vi "GUI De-Init.vi"(8 "error in (no error)":errorcluster, 10 "GUI Refs":T1, 11 "View Model":T2) -> (0 "error out":errorcluster, 3 "View Model":T2)   [LabVIEW 2017]
doc: "De - Initialize all GUI Arrays of all used modules\nMake array's size equal to 1 element values = empty"
uses:
  View Model/Controls/View Model.ctl
  View Model/Controls/Shared Model.ctl
  Error Handler/Controls/Error Model.ctl
  Error Handler/Controls/Error Event.ctl
  Error Handler/Controls/Error Type.ctl
  Controller/Controls/Controller Model.ctl
  Controller/Controls/Controller Event.ctl
  Controller/Controls/Controller Command.ctl
  Controller/Controls/Controller Overhead.ctl
  Real-Time/RT Status.ctl
  Real-Time/RT Loop Status.ctl
  Controller/Controls/Controller DAQ Data.ctl
  Controls/GUI Referencies.ctl
  Controls/AIMV_GUI_Cluster.ctl
  Controls/AOM_GUI_Cluster.ctl
  Controls/Discrete_GUI_Cluster.ctl
  GUI Init - AIMC.vi
  GUI Init - AIMV.vi
  GUI Init - AOM.vi
  GUI Init - DIM.vi
  GUI Init - DOM.vi
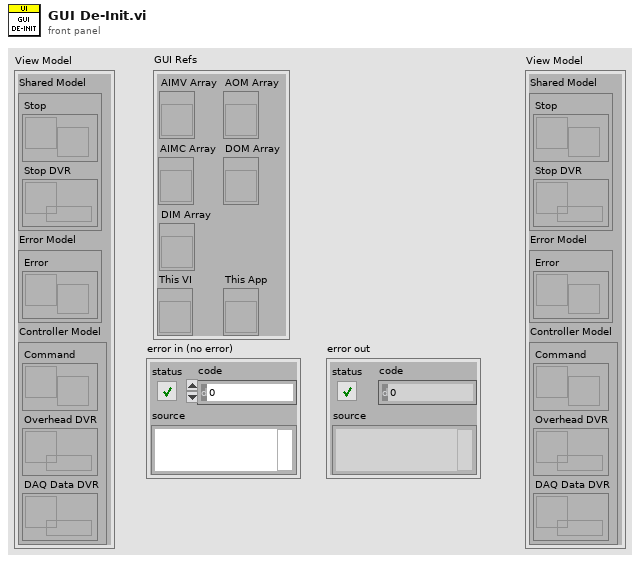
[diagram p1: front panel]
types:
  T1 = typedef "GUI Referencies.ctl" = cluster{"AIMV Array":refnum<vi>, "AIMC Array":refnum<vi>, "AOM Array":refnum<vi>, "DIM Array":refnum<vi>, "DOM Array":refnum<vi>, "This VI":refnum<vi>, "This App":refnum<vi>}
  T2 = typedef "View Model.ctl" = cluster{"Shared Model":T3, "Error Model":T4, "Controller Model":T5}
  T3 = typedef "Shared Model.ctl" = cluster{"Stop":refnum<user-event>, "Stop DVR":refnum<data-value>}
  T4 = typedef "Error Model.ctl" = cluster{"Error":refnum<user-event>}
  T5 = typedef "Controller Model.ctl" = cluster{"Command":refnum<user-event>, "Overhead DVR":refnum<data-value>, "DAQ Data DVR":refnum<data-value>}
  T6 = enum8{"Enabled", "Disabled", "Disabled and Grayed Out"}
  T7 = typedef "Controller DAQ Data.ctl" = cluster{"AOM data":dbl[], "AIMV data":dbl[], "AIMC data":dbl[], "DOM data":dbl[], "DIM data":dbl[], "AOM timestamp":dbl, "AIMV timestamp":dbl, "AIMC timestamp":dbl, "DOM timestamp":dbl, "DIM timestamp":dbl}
  T8 = typedef "AIMV_GUI_Cluster.ctl" = cluster{"Ch.name":string, "Ch.value":dbl, "Ch.range":string}
  T9 = typedef "Discrete_GUI_Cluster.ctl" = cluster{"Ch.name":string, "Ch.state":bool}
  T10 = typedef "AOM_GUI_Cluster.ctl" = cluster{"Ch.name":string, "Ch.value":dbl, "Ch.mode":enum16{"0-5 V", "+/-10 V", "0-5 mA", "4-20 mA"}}
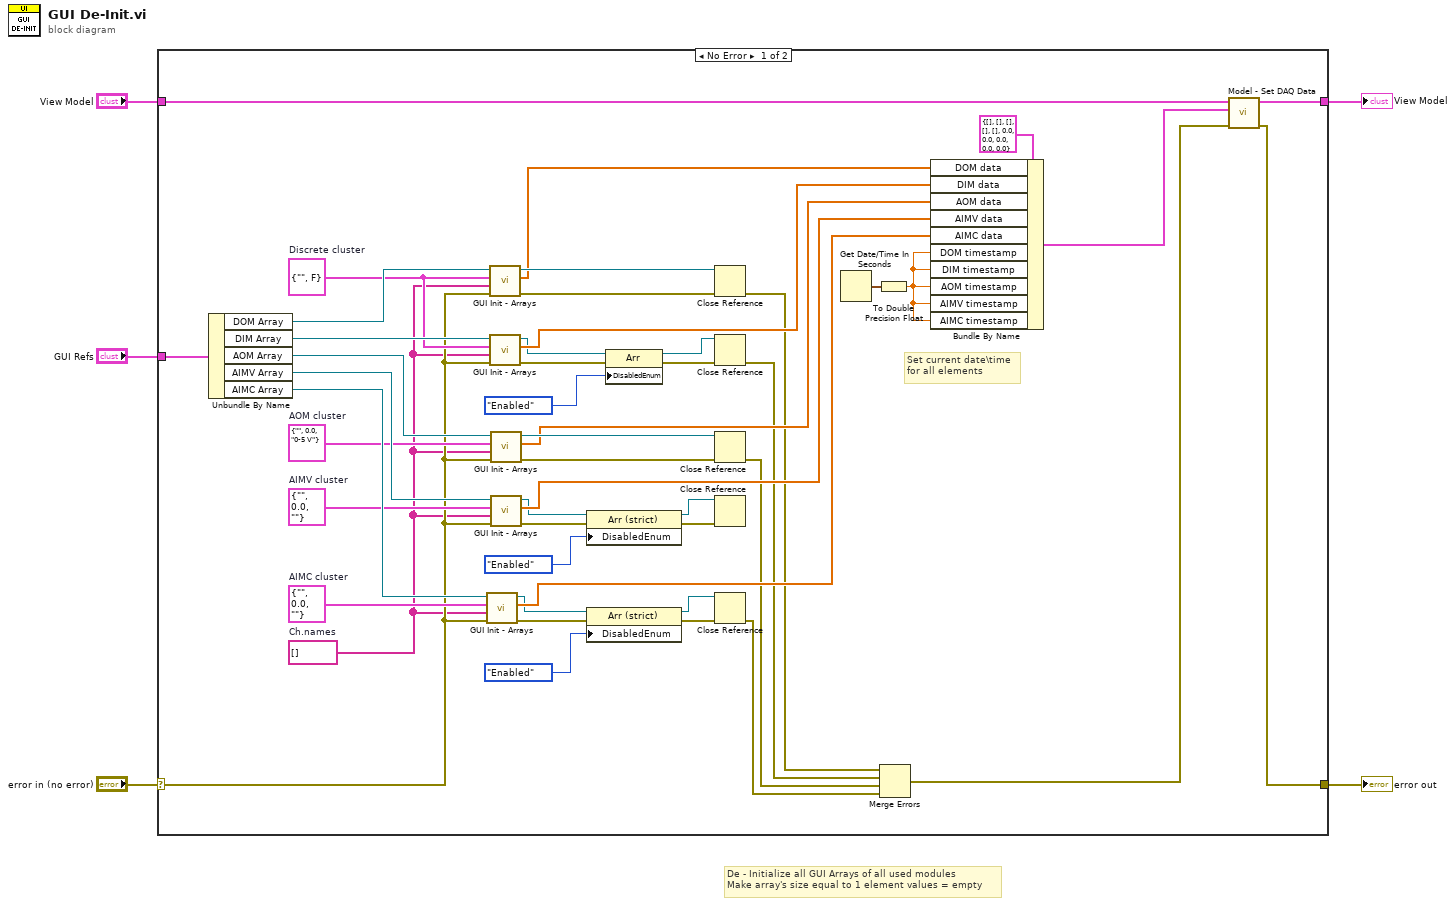
[diagram p0: block diagram]
diagram:
  # "De - Initialize all GUI Arrays of all used modules\nMake array's size equal to 1 element values = empty"
  n1 = case shown="No Error" "error in (no error)" {
    selector: "error in (no error)" -> [w43 w54]
    tunnel: [w35 w54] -> w4
    tunnel: "View Model" -> [w39 w55]
    tunnel: [w37 w55] -> w2
    tunnel: "GUI Refs" -> [w53 _]
    frame No Error {
      w45 = T8 {"Ch.name"="", "Ch.value"=0.0, "Ch.range"=""}  # AIMV cluster
      w34 = string[] []  # Ch.names
      w47 = T9 {"Ch.name"="", "Ch.state"=FALSE}  # Discrete cluster
      w46 = T10 {"Ch.name"="", "Ch.value"=0.0, "Ch.mode"=enum."0-5 V"}  # AOM cluster
      w44 = T8 {"Ch.name"="", "Ch.value"=0.0, "Ch.range"=""}  # AIMC cluster
      # "Set current date\\time\nfor all elements"
      n2 = Unbundle By Name(w53) -> ("DOM Array"=w52:refnum<vi>, "DIM Array"=w51:refnum<vi>, "AOM Array"=w50:refnum<vi>, "AIMV Array"=w49:refnum<vi>, "AIMC Array"=w48:refnum<vi>)
      n3 = call-poly "GUI Init - Arrays.vi"("error in (no error)"=w43, "Ch.names"=w34, "Cluster"=w44, "Array Ref."=w48) -> ("error out"=w18:errorcluster, "Data"=w29:dbl[], "Array Ref. out"=w9:refnum<vi>)  [unwired: 5 in]
      n4 = call-poly "GUI Init - Arrays.vi"("error in (no error)"=w43, "Ch.names"=w34, "Cluster"=w47, "Array Ref."=w52) -> ("error out"=w33:errorcluster, "Data"=w25:dbl[], "Array Ref. out"=w32:refnum<vi>)  [unwired: 5 in]
      n5 = call-poly "GUI Init - Arrays.vi"("error in (no error)"=w43, "Ch.names"=w34, "Cluster"=w47, "Array Ref."=w51) -> ("error out"=w20:errorcluster, "Data"=w26:dbl[], "Array Ref. out"=w7:refnum<vi>)  [unwired: 5 in]
      n6 = call-poly "GUI Init - Arrays.vi"("error in (no error)"=w43, "Ch.names"=w34, "Cluster"=w46, "Array Ref."=w50) -> ("error out"=w31:errorcluster, "Data"=w27:dbl[], "Array Ref. out"=w30:refnum<vi>)  [unwired: 5 in]
      n7 = call-poly "GUI Init - Arrays.vi"("error in (no error)"=w43, "Ch.names"=w34, "Cluster"=w45, "Array Ref."=w49) -> ("error out"=w16:errorcluster, "Data"=w28:dbl[], "Array Ref. out"=w11:refnum<vi>)  [unwired: 5 in]
      n8 = property class="Arr (strict)"(reference=w11, error in=w16, "DisabledEnum"=T6."Enabled" ("Disabled")) -> (reference out=w10:refnum<vi>, error out=w15:errorcluster)
      n9 = property class="Arr (strict)"(reference=w9, error in=w18, "DisabledEnum"=T6."Enabled" ("Disabled")) -> (reference out=w8:refnum<vi>, error out=w17:errorcluster)
      n10 = property class="Arr"(reference=w7, error in=w20, "DisabledEnum"=T6."Enabled" ("Disabled")) -> (reference out=w6:refnum<vi>, error out=w19:errorcluster)
      n11 = Close Reference(reference=w32, error in (no error)=w33) -> (error out=w24:errorcluster)
      n12 = Close Reference(reference=w6, error in (no error)=w19) -> (error out=w23:errorcluster)
      n13 = Close Reference(reference=w30, error in (no error)=w31) -> (error out=w22:errorcluster)
      n14 = Close Reference(reference=w10, error in (no error)=w15) -> ()  [unwired: 1 out]
      n15 = Close Reference(reference=w8, error in (no error)=w17) -> (error out=w21:errorcluster)
      n16 = Get Date/Time In Seconds() -> (seconds since 1Jan1904=w41:timestamp)
      n17 = To Double Precision Float(number=w41) -> (double precision float=w40:dbl)
      n18 = Merge Errors(w24, w23, w22, w21) -> (w36:errorcluster)
      n19 = Bundle By Name(cluster=T7 {"AOM data"=[], "AIMV data"=[], "AIMC data"=[], "DOM data"=[], "DIM data"=[], "AOM timestamp"=0.0, "AIMV timestamp"=0.0, "AIMC timestamp"=0.0, "DOM timestamp"=0.0, "DIM timestamp"=0.0} ("DAQ Data"), "DOM data"=w25, "DIM data"=w26, "AOM data"=w27, "AIMV data"=w28, "AIMC data"=w29, "DOM timestamp"=w40, "DIM timestamp"=w40, "AOM timestamp"=w40, "AIMV timestamp"=w40, "AIMC timestamp"=w40) -> (w38:T7)
      n20 = call "Model - Set DAQ Data.vi"("error in (no error)"=w36, "DAQ Data"=w38, "View Model"=w39) -> ("error out"=w35:errorcluster, "View Model"=w37:T2)  [unwired: 7 in]
    }
    frame Error {
    }
  }
  "View Model" <- w2
  "error out" <- w4
